vi "get_pixel_rate.vi"(8 "error in (no error)":errorcluster, 11 "TrajectoryAK101022Resonance in":refnum<class "TrajectoryAK101022Resonance.lvclass">) -> (0 "error out":errorcluster, 1 "pixel dwell time":dbl[unit], 2 "pixel rate":dbl[unit], 3 "TrajectoryAK101022Resonance out":refnum<class "TrajectoryAK101022Resonance.lvclass">)   [LabVIEW 2010, in "TrajectoryAK101022Resonance.lvclass"]
doc: "returns the scanning rate in Hz (i.e., pixels per second) and the pixel dwell time"
uses:
  TrajectoryAK101022Resonance.lvclass
  FPGAWrapper/GenericFPGAWrapper/GenericFPGAWrapper/GenericFPGAWrapper.lvclass
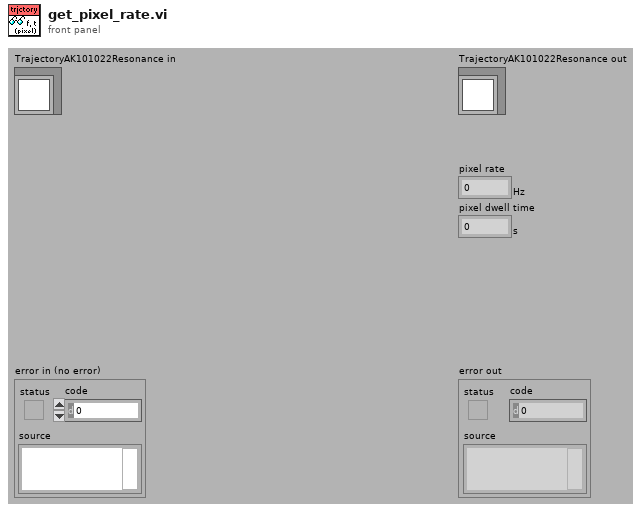
[diagram p1: front panel]
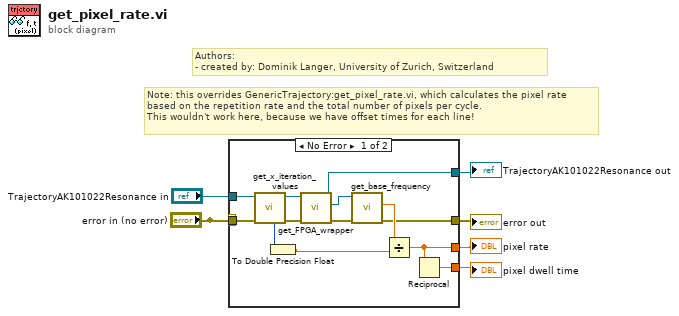
[diagram p0: block diagram]
diagram:
  # "Note: this overrides GenericTrajectory:get_pixel_rate.vi, which calculates the pixel rate based on the repetition rate and the total number of pixels per cycle.\nThis wouldn't work here, because we have offset times for each line!"
  # "Authors: \n- created by: Dominik Langer, University of Zurich, Switzerland"
  n1 = case shown="No Error" "error in (no error)" {
    selector: "error in (no error)" -> [_ w21]
    tunnel: [w8 w21] -> w6
    tunnel: "TrajectoryAK101022Resonance in" -> [w18 w20]
    tunnel: [w13 w20] -> w4
    tunnel: "error in (no error)" -> [w19 _]
    tunnel: [w9 _] -> w2
    tunnel: [w7 _] -> w1
    frame No Error {
      n2 = call-dynamic "get_x_iteration_values.vi"("error in (no error)"=w19, "TrajectoryAK101022Resonance in"=w18) -> ("error out"=w17:errorcluster, "TrajectoryAK101022Resonance out"=w16:refnum<class "TrajectoryAK101022Resonance.lvclass">, "iterations per pixel"=w12:u16)  [unwired: 4 in, 3 out]
      n3 = To Double Precision Float(number=w12) -> (double precision float=w10:dbl)
      n4 = call-dynamic "get_FPGA_wrapper.vi"("error in (no error)"=w17, "TrajectoryMG100122GenericFPGA in"=w16) -> ("error out"=w15:errorcluster, "GenericFPGAWrapper.lvclass"=w14:refnum<class "GenericFPGAWrapper.lvclass">, "TrajectoryMG100122GenericFPGA out"=w13:refnum<class "TrajectoryAK101022Resonance.lvclass">)  [unwired: 7 in]
      n5 = call-dynamic "get_base_frequency.vi"("error in (no error)"=w15, "GenericFPGAWrapper in"=w14) -> ("error out"=w8:errorcluster, "base frequency"=w11:dbl[unit])  [unwired: 7 in, 1 out]
      n6 = Divide(x=w11, y=w10) -> (x/y=w9:dbl[unit])
      n7 = Reciprocal(x=w9) -> (1/x=w7:dbl[unit])
    }
    frame Error {
    }
  }
  "error out" <- w6
  "TrajectoryAK101022Resonance out" <- w4
  "pixel rate" <- w2
  "pixel dwell time" <- w1
